vi "get modes.vi"(8 "error in (no error)":errorcluster, 11 "Camera":T3) -> (0 "error out":errorcluster, 2 "Modes":T2[](array[typedef]), 3 "Camera out":T3)   [LabVIEW 2022 SP3, in "Vision.lvlib"]
uses:
  Vision.lvlib
  camera.ctl
  camera driver.ctl
  camera mode.ctl
  <vilib>/userDefined/High Color/IMAQdx.ctl
  <vilib>/vision/driver/NI_Vision_Acquisition_Software.lvlib
panel:
  out "Video Modes":T1(array[cluster])
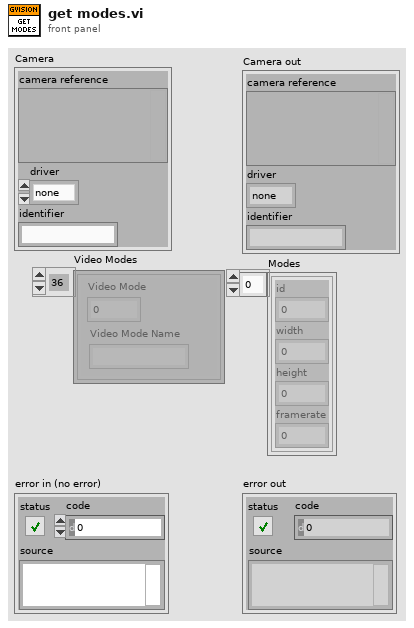
[diagram p1: front panel]
types:
  T1 = cluster{"Video Mode":u32, "Video Mode Name":string}[]
  T2 = typedef "camera mode.ctl" = cluster{"id":i32, "width":i32, "height":i32, "framerate":sgl}
  T3 = typedef "Vision.lvlib/camera.ctl" = cluster{"camera reference":variant, "driver":T4, "identifier":string}
  T4 = typedef "Vision.lvlib/camera driver.ctl" = enum16{"none", "ueye", "wmf", "imaqdx"}
  T5 = typedef "IMAQdx.ctl" = refnum<k21>
  T6 = cluster{"id":i32, "width":i32, "height":i32, "framerate":sgl}[]
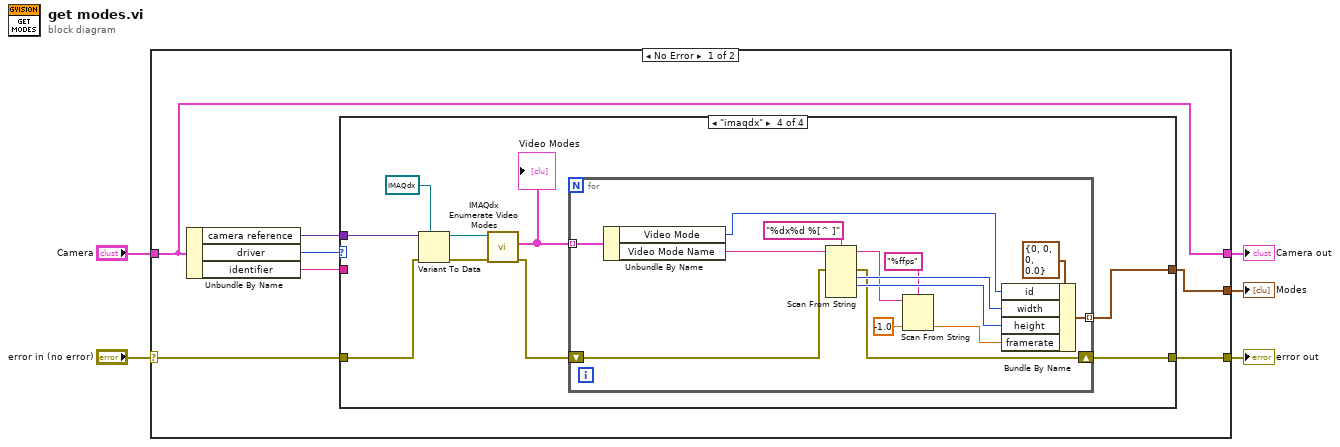
[diagram p0: block diagram]
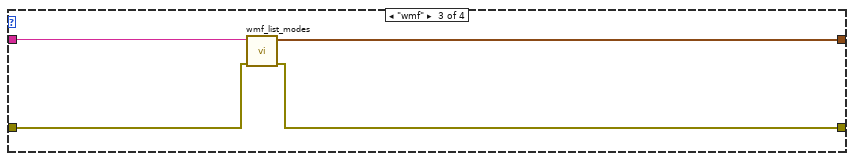
[diagram p4: hidden frame]
diagram:
  n1 = case shown="No Error" "error in (no error)" {
    selector: "error in (no error)" -> [w7 w43]
    tunnel: [w9 w43] -> w4
    tunnel: "Camera" -> [w8 w42]
    tunnel: [w8 w42] -> w2
    tunnel: [w6 _] -> w1
    frame No Error {
      n2 = Unbundle By Name(w8) -> ("camera reference"=w11:variant, "driver"=w12:T4, "identifier"=w10:string)
      n3 = case shown="\"imaqdx\"" w12 {
        tunnel: w11 -> [_ _ _ w27]
        tunnel: w10 -> [_ _ w18 _]
        tunnel: w7 -> [w13 w14 w17 w25]
        tunnel: [w13 w14 w16 w19] -> w9
        tunnel: [_ _ w15 w20] -> w6
        frame "none" {
        }
        frame "ueye" {
        }
        frame "wmf" {
          n4 = call "wmf_list_modes.vi"("error in (no error)"=w17, "camera_name"=w18) -> ("error out"=w16:errorcluster, "Modes"=w15:T6)  [unwired: 8 in]
        }
        frame "imaqdx" {
          n5 = Variant To Data(error in=w25, type=T5 refnum ("Session In"), Variant=w27) -> (data=w23:T5, error out=w24:errorcluster)
          n6 = call <vilib>:"IMAQdx Enumerate Video Modes.vi"("error in"=w24, "Session In"=w23) -> ("error out"=w21:errorcluster, "Video Modes"=w22:T1)  [unwired: 6 in, 2 out]
          "Video Modes" <- w22
          n7 = for {
            tunnel: w22 -> [w41] mode=indexing
            shift-right: [w32] -> w19
            shift-left: w21 -> [w38]
            tunnel: [w33] -> w20 mode=indexing
            n8 = Unbundle By Name(w41) -> ("Video Mode"=w36:u32, "Video Mode Name"=w40:string)
            n9 = Scan From String(format string="%dx%d %[^ ]", input string=w40, error in=w38) -> (remaining string=w31:string, error out=w32:errorcluster, output 1=w35:i32, output 2=w34:i32)  [unwired: 5 in, 1 out]
            n10 = Scan From String(format string="%ffps", input string=w31, default 1=-1.0 ("default value 1")) -> (output 1=w28:dbl)  [unwired: 2 in, 3 out]
            n11 = Bundle By Name(cluster=T2 {"id"=0, "width"=0, "height"=0, "framerate"=0.0} ("Cluster"), "id"=w36, "width"=w35, "height"=w34, "framerate"=w28) -> (w33:T2)
          }
        }
      }
    }
    frame Error {
    }
  }
  "error out" <- w4
  "Camera out" <- w2
  "Modes" <- w1
